vi "testEmptyElement.vi"(8 "error in (no error)":errorcluster, 11 "reference in":refnum<class "EasyXMLTest.lvclass">) -> (0 "error out":errorcluster, 3 "reference in":refnum<class "EasyXMLTest.lvclass">)   [LabVIEW 2013, in "EasyXMLTest.lvclass"]
uses:
  EasyXMLTest.lvclass
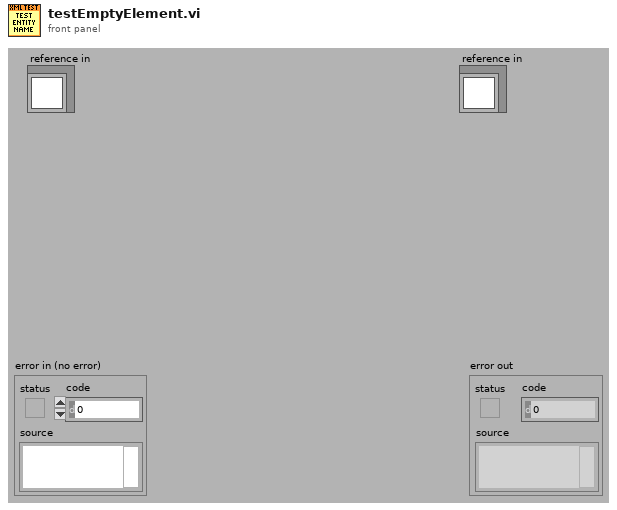
[diagram p1: front panel]
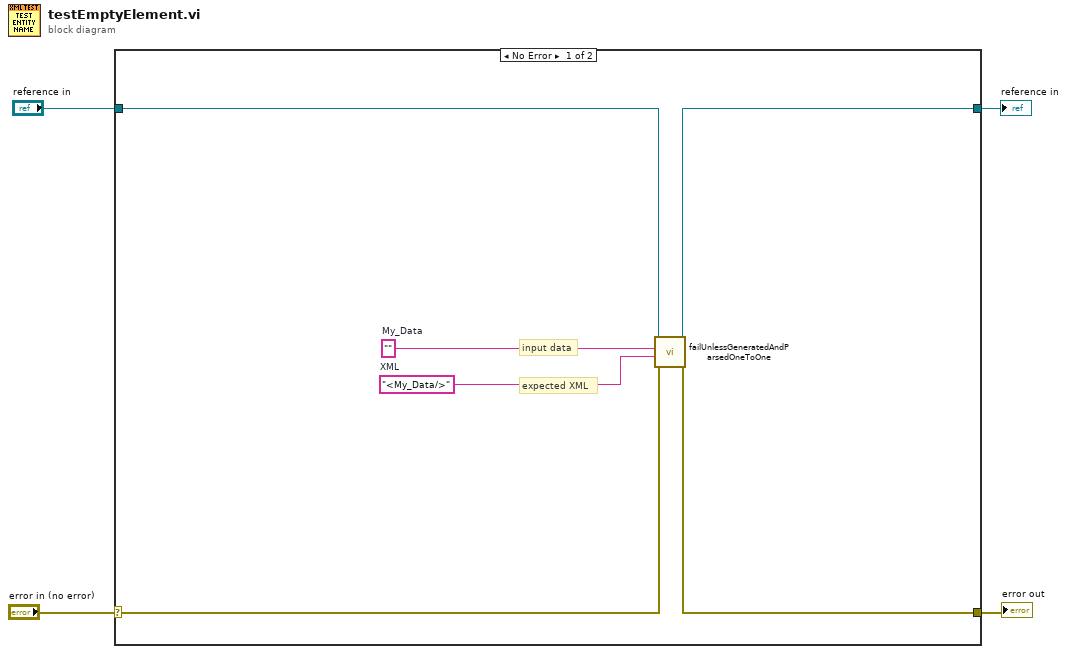
[diagram p0: block diagram]
diagram:
  n1 = case shown="No Error" "error in (no error)" {
    selector: "error in (no error)" -> [w5 w12]
    tunnel: [w10 w12] -> w3
    tunnel: [w8 w11] -> w1
    tunnel: "reference in" -> [w9 w11]
    frame No Error {
      w6 = "<My_Data/>"  # XML
      w7 = ""  # My_Data
      # "expected XML"
      # "input data"
      n2 = call "failUnlessGeneratedAndParsedOneToOne.vi"("error in"=w5, "XML String"=w6, "Data"=w7, "EasyXMLTest in"=w9) -> ("error out"=w10:errorcluster, "EasyXMLTest out"=w8:refnum<class "EasyXMLTest.lvclass">)  [unwired: 4 in, 2 out]
    }
    frame Error {
    }
  }
  "error out" <- w3
  "reference in" <- w1
